vi "comm lock.vi"(8 "error in (no error)":errorcluster, 10 "Timeout (-1:infinitive)":i32, 11 "Comm Handle":u64) -> (0 "error out":errorcluster, 3 "dup Comm Handle":u64)   [LabVIEW 2009, in "lvserial.lvlib"]
doc: "Locks the serial port."
uses:
  lvserial.lvlib
  x64/Release/lvserial.dll
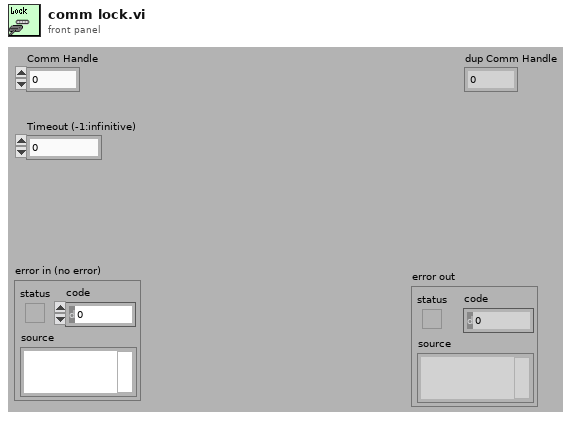
[diagram p1: front panel]
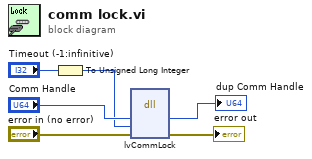
[diagram p0: block diagram]
diagram:
  n1 = To Unsigned Long Integer(number="Timeout (-1:infinitive)") -> (unsigned 32bit integer=w1:u32)
  n2 = dll-call lib="C:/Users/Admin/Desktop/lvserial_source_1-2-13/x64/Release/lvserial.dll" fn="lvCommLock"("hComm"="Comm Handle", "ulTimeout"=w1, "error"="error in (no error)") -> ("hComm"=→"dup Comm Handle":u64, "error"=→"error out":errorcluster)  [unwired: 4 in, 3 out]
